vi "Utility Example.vi"() -> ()   [LabVIEW 2010]
doc: "This example shows how to use VIs in the utility palette."
uses:
  Type Defs/File Format.ctl
  Type Defs/Single Tag.ctl
  Type Defs/Data Types.ctl
  Type Defs/Tag Grouping set.ctl
  FGVs/Tag Memory.vi
  Current Value Table.lvlib
panel:
  out "error out":errorcluster
  in  "Path for Full CVT":path=path "C:/Users/Public/Documents/FullCVT.xml"
  in  "Path for Mission Critical Data Group":path=path "C:/Users/Public/Documents/MissionCriticalGroup.xml"
  out "Tag 2 Description":string
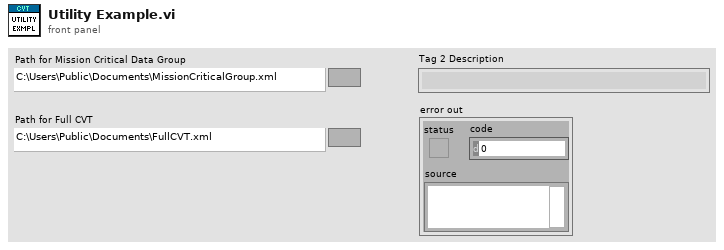
[diagram p1: front panel]
types:
  T1 = typedef "Current Value Table.lvlib/File Format.ctl" = cluster{"Tags":T2[], "Group Listings":T4[]}
  T2 = typedef "Current Value Table.lvlib/Single Tag.ctl" = cluster{"Data Type":T3, "Name":string, "Value":string, "Description":string}
  T3 = typedef "Current Value Table.lvlib/Data Types.ctl" = enum16{"Double", "Single", "I64", "I32", "I16", "I8", "U64", "U32", "U16", "U8", "String", "Boolean", "Array of U8", "Array of U16", "Array of U32", "Array of U64", "Array of I64", "Array of I32", "Array of I16", "Array of I8", "Array of Double", "Array of Single", "Array of Boolean", "Array of String"}
  T4 = typedef "Current Value Table.lvlib/Tag Grouping set.ctl" = cluster{"Group":string, "Tag Names":string[]}
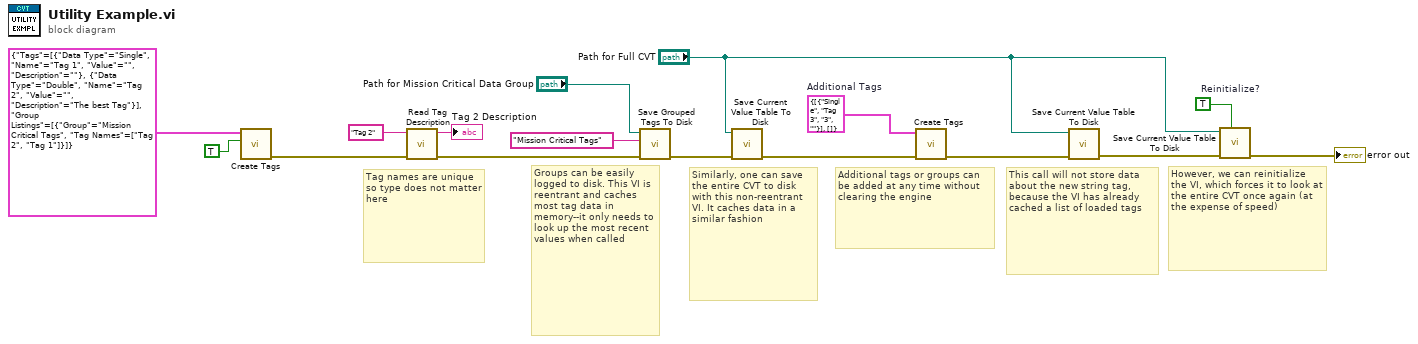
[diagram p0: block diagram]
diagram:
  w3 = TRUE  # Reinitialize?
  w6 = T1 {"Tags"=[{"Data Type"=enum."Single", "Name"="Tag 3", "Value"="3", "Description"=""}], "Group Listings"=[]}  # Additional Tags
  # "However, we can reinitialize the VI, which forces it to look at the entire CVT once again (at the expense of speed)"
  # "This call will not store data about the new string tag, because the VI has already cached a list of loaded tags"
  # "Additional tags or groups can be added at any time without clearing the engine"
  # "Similarly, one can save the entire CVT to disk with this non-reentrant VI. It caches data in a similar fashion"
  # "Groups can be easily logged to disk. This VI is reentrant and caches most tag data in memory--it only needs to look up the most recent values when called"
  # "Tag names are unique so type does not matter here"
  n1 = call "Create Tags.vi"("Clear Table? (F)"=TRUE ("Clear Engine?"), "CVT Tags to Create"=T1 {"Tags"=[{"Data Type"=enum."Single", "Name"="Tag 1", "Value"="", "Description"=""}, {"Data Type"=enum."Double", "Name"="Tag 2", "Value"="", "Description"="The best Tag"}], "Group Listings"=[{"Group"="Mission Critical Tags", "Tag Names"=["Tag 2", "Tag 1"]}]} ("CVT File Data")) -> ("error out"=w13:errorcluster)  [unwired: 9 in]
  n2 = call "Read Tag Description.vi"("error in (no error)"=w13, "Tag Name"="Tag 2") -> ("error out"=w11:errorcluster, "Description"=→"Tag 2 Description":string)  [unwired: 8 in]
  n3 = call "Save Grouped Tags To Disk.vi"("error in (no error)"=w11, "Group"="Mission Critical Tags", "XML File Path"="Path for Mission Critical Data Group") -> ("error out"=w10:errorcluster)  [unwired: 8 in]
  n4 = call "Save Current Value Table To Disk.vi"("error in (no error)"=w10, "XML File Path"="Path for Full CVT") -> ("error out"=w7:errorcluster)  [unwired: 9 in]
  n5 = call "Create Tags.vi"("error in (no error)"=w7, "CVT Tags to Create"=w6) -> ("error out"=w5:errorcluster)  [unwired: 9 in]
  n6 = call "Save Current Value Table To Disk.vi"("error in (no error)"=w5, "XML File Path"="Path for Full CVT") -> ("error out"=w4:errorcluster)  [unwired: 9 in]
  n7 = call "Save Current Value Table To Disk.vi"("Force Lookup? (F)"=w3, "error in (no error)"=w4, "XML File Path"="Path for Full CVT") -> ("error out"=→"error out":errorcluster)  [unwired: 8 in]
